vi "名称更新(-1)-8.6.vi"(3 "输入":path) -> (0 "名称":string, 1 "输出":path)   [LabVIEW 2013]
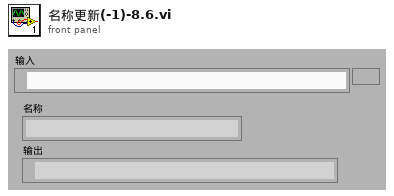
[diagram p1: front panel]
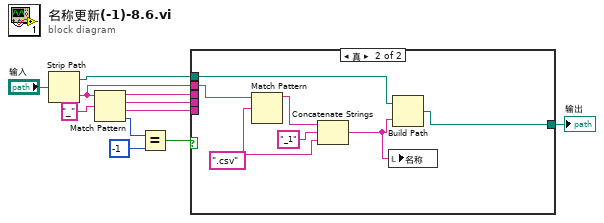
[diagram p0: block diagram]
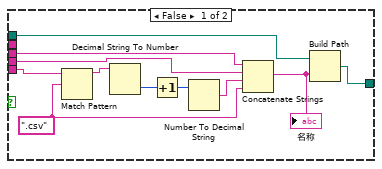
[diagram p2: hidden frame]
diagram:
  n1 = Strip Path(path="输入") -> (stripped path=w6:path, name=w7:string)
  n2 = Match Pattern(string=w7, regular expression="_" ("正则表达式")) -> (before substring=w4:string, match substring=w3:string, after substring=w5:string, offset past match=w10:i32)  [unwired: 1 out]
  n3 = Equal?(x=w10, y=-1) -> (x = y?=w8:bool)
  n4 = case shown="真" w8 {
    tunnel: w7 -> [_ w28]
    tunnel: w6 -> [w13 w25]
    tunnel: [w12 w24] -> w1
    tunnel: w5 -> [w16 _]
    tunnel: w4 -> [w20 _]
    tunnel: w3 -> [w19 _]
    frame False {
      w15 = ".csv" ("正则表达式")
      n5 = Match Pattern(string=w16, regular expression=w15) -> (before substring=w17:string)  [unwired: 4 out]
      n6 = Decimal String To Number(string=w17) -> (number=w22:i32)  [unwired: 3 out]
      n7 = Increment(x=w22) -> (x+1=w21:i32)
      n8 = Number To Decimal String(number=w21) -> (decimal integer string=w18:string)  [unwired: 1 out]
      n9 = Concatenate Strings(w20, w19, w18, w15) -> (w14:string)
      "名称" <- w14
      n10 = Build Path(base path=w13, name or relative path=w14) -> (appended path=w12:path)
    }
    frame True {
      w26 = ".csv" ("正则表达式")
      n11 = Match Pattern(string=w28, regular expression=w26) -> (before substring=w27:string)  [unwired: 4 out]
      n12 = Concatenate Strings(w27, "_1" ("正则表达式"), w26) -> (w23:string)
      n13 = local write "名称"(w23) -> ()
      n14 = Build Path(base path=w25, name or relative path=w23) -> (appended path=w24:path)
    }
  }
  "输出" <- w1
